vi "Gather Statistics.vi"(10 "JSON Statistics":refnum<class "JSON Statistics.lvclass">, 11 "JSON Value In":refnum<class "JSON Value.lvclass">) -> (3 "JSON Statistic or Object":refnum<class "JSON Value.lvclass">)   [LabVIEW 2020, in "Library Commun.lvlib" / "JSON Statistics.lvclass"]
uses:
  JSON Statistics.lvclass
  JSON Value/JSON Value.lvclass
  C:/Users/ngarcin/OneDrive - Altyor/Standard TB/Class/JSON API/JSON Value/JSON Value.lvclass
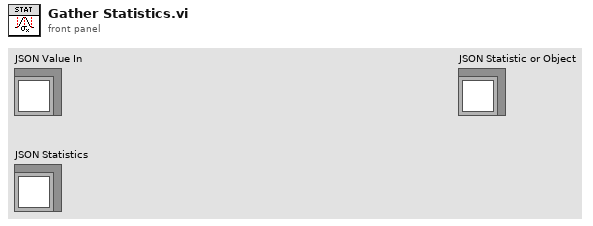
[diagram p1: front panel]
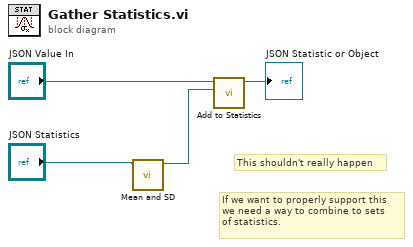
[diagram p0: block diagram]
diagram:
  # "If we want to properly support this\nwe need a way to combine to sets\nof statistics."
  # "This shouldn't really happen"
  n1 = call-dynamic "Mean and SD.vi"("JSON Statistics in"="JSON Statistics") -> ("JSON Value"=w1:refnum<class "JSON Value.lvclass">)  [unwired: 8 in, 2 out]
  n2 = call-dynamic "Add to Statistics.vi"("Non Object"=w1, "JSON Value In"="JSON Value In") -> ("JSON Statistics out"=→"JSON Statistic or Object":refnum<class "JSON Statistics.lvclass">)  [unwired: 9 in]
